vi "Select Data Subset From Loaded Data.vi"(5 "CycleAngle?":T2, 6 "Memory Size as number":i32, 7 "MissingTeeth":dbl, 8 "ReverseData":bool, 9 "Offset":i32, 10 "Data Selection Method":T1, 11 "Signal":dbl[](array[numeric])) -> (1 "Selected Length":i32, 2 "Selected Offset":i32, 3 "Resampled Data":dbl[](array[numeric]))   [LabVIEW 2015, in "Data Replay File.lvlib"]
uses:
  Data Replay File.lvlib
  AngleReference.ctl
  Data Replay Data Selection Method.ctl
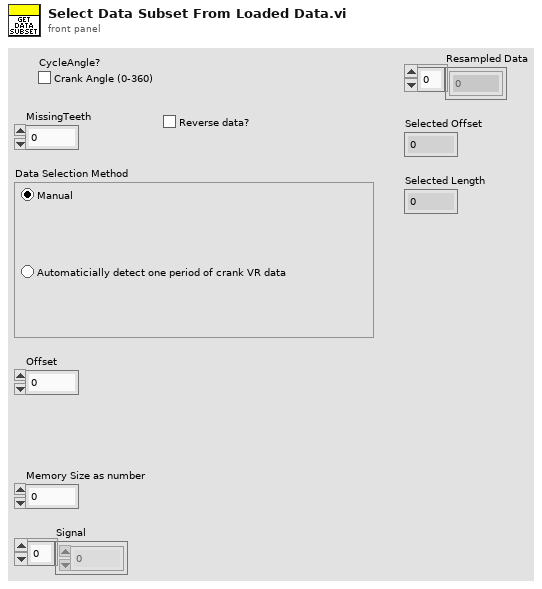
[diagram p1: front panel]
types:
  T1 = typedef "Data Replay Data Selection Method.ctl" = enum32{"Manual", "AutoVRCrank"}
  T2 = typedef "AngleReference.ctl" = bool
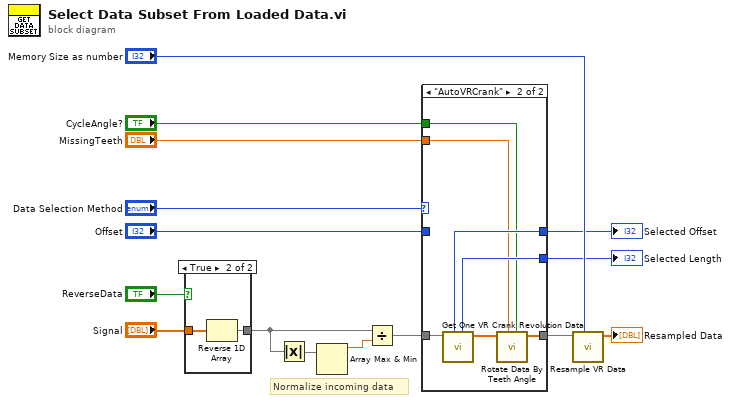
[diagram p0: block diagram]
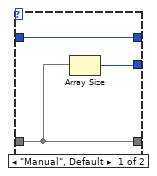
[diagram p3: hidden frame]
diagram:
  # "Normalize incoming data"
  n1 = case shown="True" "ReverseData" {
    tunnel: "Signal" -> [w16 w18]
    tunnel: [w16 w17] -> w2
    frame False {
    }
    frame True {
      n2 = Reverse 1D Array(array=w18) -> (reversed array=w17:dbl[])
    }
  }
  n3 = Absolute Value(x=w2) -> (abs(x)=w3:dbl[])
  n4 = Array Max & Min(array=w3) -> (max value=w4:dbl)  [unwired: 3 out]
  n5 = Divide(x=w2, y=w4) -> (x/y=w7:dbl[])
  n6 = case shown="\"AutoVRCrank\"" "Data Selection Method" {
    tunnel: w7 -> [w20 w28]
    tunnel: [w21 w27] -> w8
    tunnel: [w19 w26] -> w9
    tunnel: "Offset" -> [w21 _]
    tunnel: "MissingTeeth" -> [_ w24]
    tunnel: "CycleAngle?" -> [_ w23]
    tunnel: [w20 w22] -> w13
    frame "Manual", Default {
      n7 = Array Size(array=w20) -> (size(s)=w19:i32)
    }
    frame "AutoVRCrank" {
      n8 = call "Get One VR Crank Revolution Data.vi"("Data In"=w28) -> ("One VR Crank Period"=w25:dbl[], "Selected Length"=w26:i32, "Selected Offset"=w27:i32)  [unwired: 8 in]
      n9 = call "Rotate Data By Teeth Angle.vi"("CycleAngle?"=w23, "Missing Tooth Angle"=w24, "One VR Crank Period"=w25) -> ("Rotated to desired angle"=w22:dbl[])  [unwired: 8 in]
    }
  }
  "Selected Length" <- w9
  "Selected Offset" <- w8
  n10 = call "Resample VR Data.vi"("Memory Size"="Memory Size as number", "Data In"=w13) -> ("Resampled Data"=→"Resampled Data":dbl[])  [unwired: 9 in]
